vi "InternalResource.vi"(7 "action":T1, 10 "count":i32, 11 "name":string) -> (2 "wait list":string[](array[string]), 3 "active list":string[](array[string]))   [LabVIEW 2017, in "McsaResourceSchedulerLR.lvlib"]
uses:
  <vilib>/addons/InsightCM/Devices/Shared/Mcsa/McsaResourceSchedulerLR/McsaResourceSchedulerLR.lvlib
  <vilib>/addons/InsightCM/Devices/Shared/Mcsa/McsaResourceSchedulerLR/controls/InternalAction.ctl
panel:
  out "error out":errorcluster
  in  "error in (no error)":errorcluster
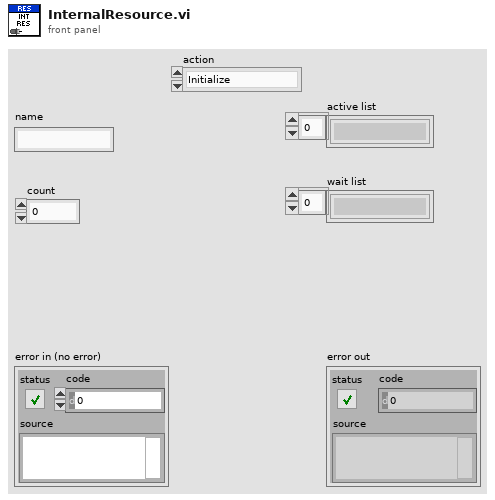
[diagram p1: front panel]
types:
  T1 = typedef "McsaResourceSchedulerLR.lvlib/InternalAction.ctl" = enum16{"Initialize", "Register", "Unregister", "Get"}
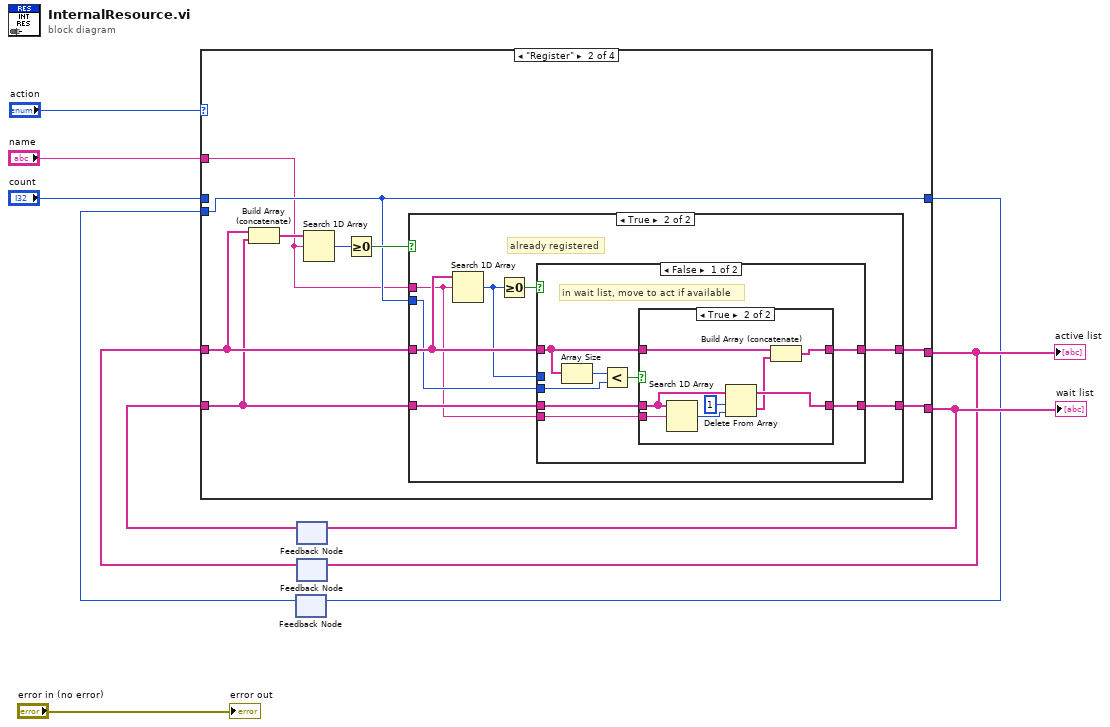
[diagram p0: block diagram]
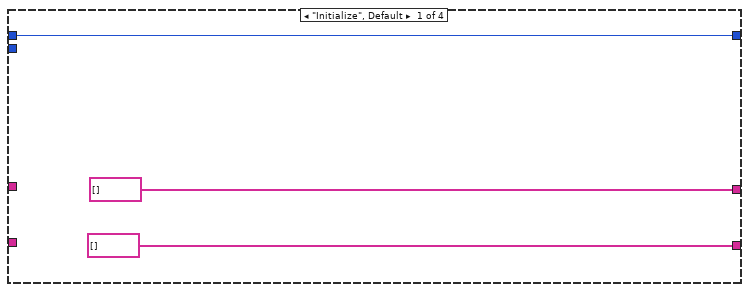
[diagram p2: hidden frame]
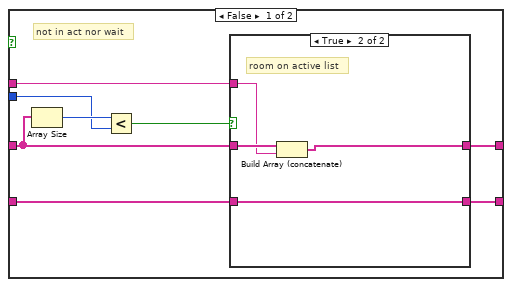
[diagram p3: hidden frame]
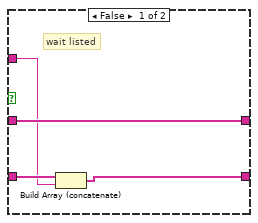
[diagram p4: hidden frame]
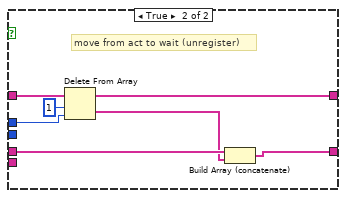
[diagram p6: hidden frame]
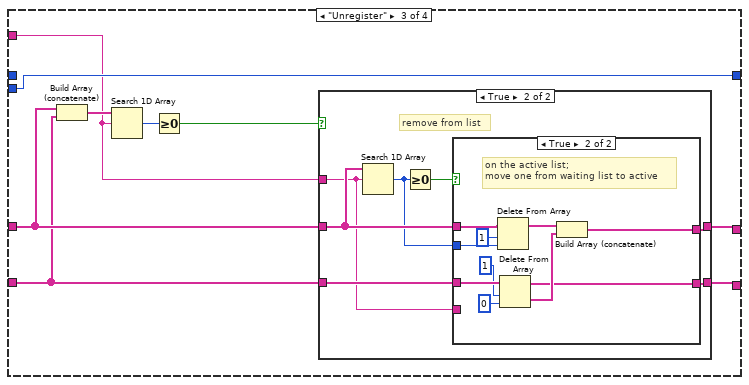
[diagram p7: hidden frame]
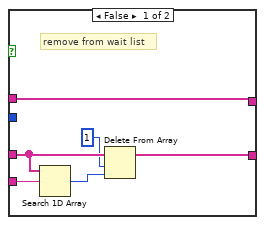
[diagram p9: hidden frame]
diagram:
  n1 = feedback #1() -> (w2:i32)  [unwired: 1 in]
  n2 = feedback #2() -> (w7:string[])  [unwired: 1 in]
  n3 = feedback #3() -> (w5:string[])  [unwired: 1 in]
  n4 = case shown="\"Register\"" "action" {
    tunnel: [string[] [] w18 w75 w107] -> w6
    tunnel: [string[] [] w16 w73 w106] -> w8
    tunnel: w7 -> [_ w17 w74 w106]
    tunnel: w5 -> [_ w19 w76 w107]
    tunnel: [w11 w15 w80 w108] -> w3
    tunnel: "count" -> [w11 _ _ _]
    tunnel: w2 -> [_ w15 w80 w108]
    tunnel: "name" -> [_ w14 w72 _]
    frame "Initialize", Default {
    }
    frame "Register" {
      n5 = Build Array (concatenate)(w19, w17) -> (w22:string[])
      n6 = Search 1D Array(1D array=w22, element=w14) -> (index of element=w21:i32)  [unwired: 1 in]
      n7 = Greater Or Equal To 0?(x=w21) -> (x >= 0?=w20:bool)
      n8 = case shown="True" w20 {
        tunnel: w19 -> [w27 w45]
        tunnel: [w24 w42] -> w18
        tunnel: w17 -> [w26 w44]
        tunnel: [w23 w41] -> w16
        tunnel: w15 -> [w29 w40]
        tunnel: w14 -> [w25 w39]
        frame False {
          # "not in act nor wait"
          n9 = Array Size(array=w27) -> (size(s)=w30:i32)
          n10 = Less?(x=w30, y=w29) -> (x < y?=w28:bool)
          n11 = case shown="True" w28 {
            tunnel: w27 -> [w34 w38]
            tunnel: w26 -> [w33 w35]
            tunnel: w25 -> [w32 w37]
            tunnel: [w34 w36] -> w24
            tunnel: [w31 w35] -> w23
            frame False {
              # "wait listed"
              n12 = Build Array (concatenate)(w33, w32) -> (w31:string[])
            }
            frame True {
              # "room on active list"
              n13 = Build Array (concatenate)(w38, w37) -> (w36:string[])
            }
          }
        }
        frame True {
          # "already registered"
          n14 = Search 1D Array(1D array=w45, element=w39) -> (index of element=w43:i32)  [unwired: 1 in]
          n15 = Greater Or Equal To 0?(x=w43) -> (x >= 0?=w46:bool)
          n16 = case shown="False" w46 {
            tunnel: w45 -> [w50 w71]
            tunnel: w44 -> [w51 w67]
            tunnel: w43 -> [_ w69]
            tunnel: [w49 w68] -> w42
            tunnel: [w47 w65] -> w41
            tunnel: w40 -> [w53 _]
            tunnel: w39 -> [w48 _]
            frame False {
              # "in wait list, move to act if available"
              n17 = Array Size(array=w50) -> (size(s)=w54:i32)
              n18 = Less?(x=w54, y=w53) -> (x < y?=w52:bool)
              n19 = case shown="True" w52 {
                tunnel: w51 -> [w55 w61]
                tunnel: w50 -> [w56 w64]
                tunnel: [w56 w63] -> w49
                tunnel: w48 -> [_ w62]
                tunnel: [w55 w60] -> w47
                frame False {
                }
                frame True {
                  n20 = Search 1D Array(1D array=w61, element=w62) -> (index of element=w58:i32)  [unwired: 1 in]
                  n21 = Delete From Array(array=w61, length=1, index=w58) -> (deleted portion=w59:string[], array with subset deleted=w60:string[])
                  n22 = Build Array (concatenate)(w64, w59) -> (w63:string[])
                }
              }
            }
            frame True {
              # "move from act to wait (unregister)"
              n23 = Delete From Array(array=w71, length=1, index=w69) -> (deleted portion=w66:string[], array with subset deleted=w68:string[])
              n24 = Build Array (concatenate)(w67, w66) -> (w65:string[])
            }
          }
        }
      }
    }
    frame "Unregister" {
      n25 = Build Array (concatenate)(w76, w74) -> (w79:string[])
      n26 = Search 1D Array(1D array=w79, element=w72) -> (index of element=w78:i32)  [unwired: 1 in]
      n27 = Greater Or Equal To 0?(x=w78) -> (x >= 0?=w77:bool)
      n28 = case shown="True" w77 {
        tunnel: w76 -> [w82 w88]
        tunnel: [w82 w85] -> w75
        tunnel: w74 -> [w81 w86]
        tunnel: [w81 w84] -> w73
        tunnel: w72 -> [_ w83]
        frame False {
          # "not registered"
        }
        frame True {
          # "remove from list"
          n29 = Search 1D Array(1D array=w88, element=w83) -> (index of element=w87:i32)  [unwired: 1 in]
          n30 = Greater Or Equal To 0?(x=w87) -> (x >= 0?=w89:bool)
          n31 = case shown="True" w89 {
            tunnel: w88 -> [w95 w105]
            tunnel: w87 -> [_ w104]
            tunnel: w86 -> [w93 w103]
            tunnel: [w95 w96] -> w85
            tunnel: [w91 w100] -> w84
            tunnel: w83 -> [w94 _]
            frame False {
              # "remove from wait list"
              n32 = Search 1D Array(1D array=w93, element=w94) -> (index of element=w92:i32)  [unwired: 1 in]
              n33 = Delete From Array(array=w93, length=1, index=w92) -> (array with subset deleted=w91:string[])  [unwired: 1 out]
            }
            frame True {
              # "on the active list;\nmove one from waiting list to active"
              n34 = Delete From Array(array=w105, length=1, index=w104) -> (array with subset deleted=w98:string[])  [unwired: 1 out]
              n35 = Delete From Array(array=w103, length=1, index=0) -> (deleted portion=w101:string[], array with subset deleted=w100:string[])
              n36 = Build Array (concatenate)(w98, w101) -> (w96:string[])
            }
          }
        }
      }
    }
    frame "Get" {
    }
  }
  "active list" <- w6
  "wait list" <- w8
  n37 = feedback-in #1(w3) -> ()
  n38 = feedback-in #2(w8) -> ()
  n39 = feedback-in #3(w6) -> ()
  "error out" <- "error in (no error)"
